vi "New Report Schema and Table Create.vi"(8 "error in":errorcluster, 11 "Schema":string="eDCU_LTT_RESULTS") -> (0 "error out":errorcluster)   [LabVIEW 2023]
uses:
  Database/SQL Public VI/Control/DB Options.ctl
  Database/Database.lvclass
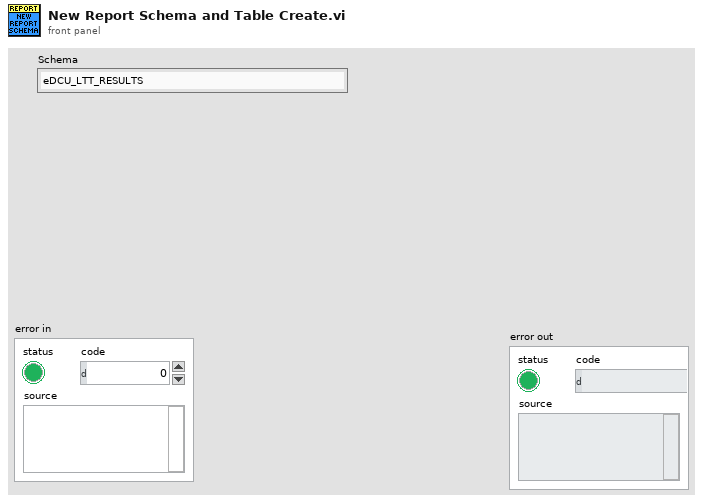
[diagram p1: front panel]
types:
  T1 = typedef "HardwareAbstractionLayer_LVOOP.lvlib/Database.lvclass/DB Options.ctl" = enum16{"Init", "Select Data", "Insert Data", "Update Data", "Delete Data", "Execute Query", "Create Schema", "Create Table", "List Tables", "List Columns", "Close"}
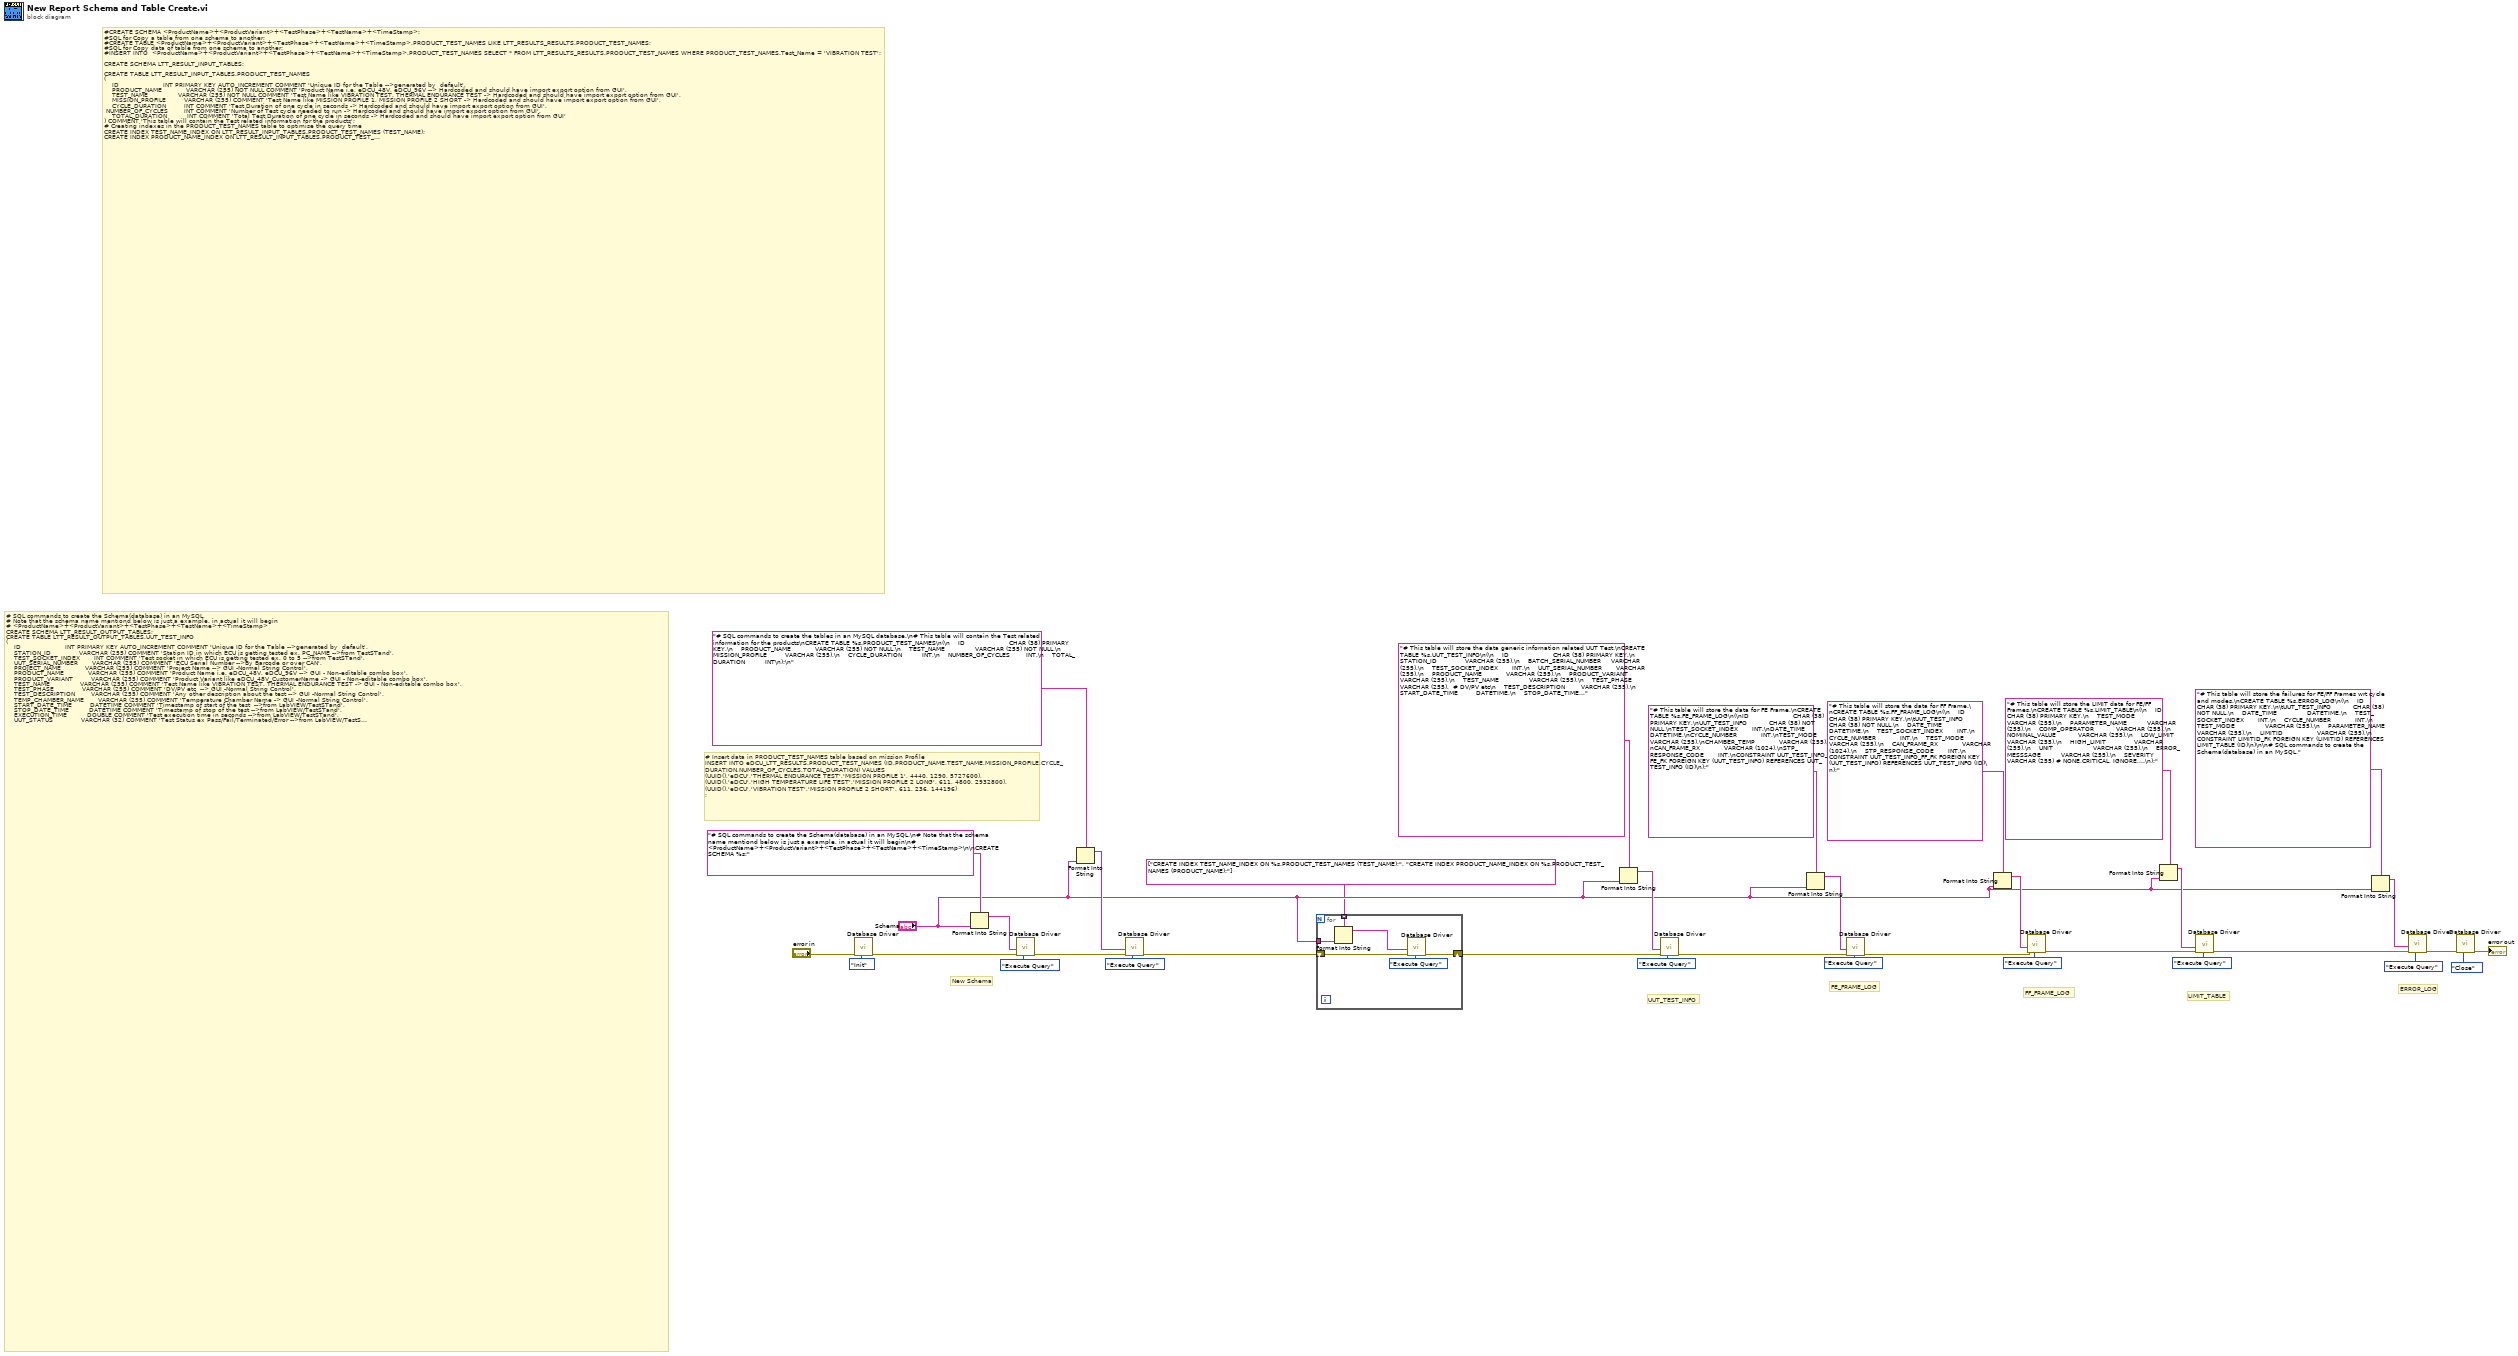
[diagram p0: block diagram]
diagram:
  # "# SQL commands to create the Schema(database) in an MySQL.\n# Note that the schema name mentiond below is just a example, in actual it will begin\n# <ProductName>+<ProductVariant>+<TestPhase>+<TestName>+<TimeStamp>\nCREATE SCHEMA LTT_RESULT_OUTPUT_TABLES;\nCREATE TABLE LTT_RESULT_OUTPUT_TABLES.UUT_TEST_INFO\n(\n    ID                      INT PRIMARY KEY AUTO_INCREMENT COMMENT 'Unique ID for the Table -->generated by  default',\n    STATION_ID              VARCHAR (255) COMMENT 'Station ID in which ECU is getting tested ex. PC_NAME -->from TestSTand',\n    TEST_SOCKET_INDEX       INT COMMENT 'Test socket in which ECU is getting tested ex. 0 to 5 -->from TestSTand',\n    UUT_SERIAL_NUMBER       VARCHAR (255) COMMENT 'ECU Serial Number -->By Barcode or over CAN',\n    PROJECT_NAME            VARCHAR (255) COMMENT 'Project Name --> GUI -Normal String Control',\n    PRODUCT_NAME            VARCHAR (255) COMMENT 'Product Name i.e. eDCU_48V, eDCU_96V --> GUI - Non-editable combo box',\n    PRODUCT_VARIANT         VARCHAR (255) COMMENT 'Product Variant like eDCU_48V_CustomerName -> GUI - Non-editable combo box',\n    TEST_NAME               VARCHAR (255) COMMENT 'Test Name like VIBRATION TEST, THERMAL ENDURANCE TEST -> GUI - Non-editable combo box',\n    TEST_PHASE              VARCHAR (255) COMMENT 'DV/PV etc  --> GUI -Normal String Control',\n    TEST_DESCRIPTION        VARCHAR (255) COMMENT 'Any other description about the test --> GUI -Normal String Control',\n    TEMP_CHAMBER_NAME       VARCHAR (255) COMMENT 'Temperature Chamber Name -> GUI -Normal String Control',\n    START_DATE_TIME         DATETIME COMMENT 'Timestamp of start of the test  -->from LabVIEW/TestSTand',\n    STOP_DATE_TIME          DATETIME COMMENT 'Timestamp of stop of the test -->from LabVIEW/TestSTand',\n    EXECUTION_TIME          DOUBLE COMMENT 'Test execution time in seconds -->from LabVIEW/TestSTand',\n    UUT_STATUS              VARCHAR (32) COMMENT 'Test Status ex Pass/Fail/Terminated/Error -->from LabVIEW/TestSTand',\n    UUT_ERROR_CODE          INT COMMENT 'Error code in case of any error -->from LabVIEW/TestSTand',\n    UUT_ERROR_MESSAGE       VARCHAR (255) COMMENT 'Error Description in case of any error -->from LabVIEW/TestSTand'\n) COMMENT 'This table will store the data generic infornation related UUT Test';\n \nCREATE TABLE LTT_RESULT_OUTPUT_TABLES.FE_FRAME_LOG\n(\n    ID                      INT PRIMARY KEY AUTO_INCREMENT COMMENT 'Unique ID for the Table -->generated by  default',\n\tUUT_TEST_INFO           INT NOT NULL COMMENT 'ID from UUT_TEST_INFO table for that perticular test --> MySQL DB',\n    TEST_SOCKET_INDEX       INT COMMENT 'Test socket in which ECU is getting tested ex. 0 to 5 -->from TestSTand',\n    DATE_TIME               DATETIME COMMENT 'Timestamp when the Frame is received -->from LabVIEW/TestSTand',\n    CYCLE_NUMBER            INT COMMENT 'Current Test Cycle Number of Mission Profile -->from LabVIEW/TestSTand',\n    TEST_MODE               VARCHAR (255) COMMENT 'Current Test Mode of Mission Profile -->from LabVIEW/TestSTand',\n    CHAMBER_TEMP            VARCHAR (255) COMMENT 'Current Temperature of Chamber -->from LabVIEW/TestSTand',\n    CAN_FRAME_RX            VARCHAR (1024) COMMENT 'Raw CAN Frame received over STP -->from LabVIEW/TestSTand',\n    STP_RESPONSE_CODE       INT COMMENT 'STP Response code or Status  received over STP -->from LabVIEW/TestSTand',\n    CONSTRAINT UUT_TEST_INFO_FE_FK FOREIGN KEY (UUT_TEST_INFO) REFERENCES UUT_TEST_INFO (ID)\n) COMMENT 'This table will store the data for FE Frame';\n\n\nCREATE TABLE LTT_RESULT_OUTPUT_TABLES.FF_FRAME_LOG\n(\n    ID                      INT PRIMARY KEY AUTO_INCREMENT COMMENT 'Unique ID for the Table -->generated by  default',\n\tUUT_TEST_INFO           INT NOT NULL COMMENT 'ID from UUT_TEST_INFO table for that perticular test --> MySQL DB',\n\tTEST_SOCKET_INDEX       INT COMMENT 'Test socket in which ECU is getting tested ex. 0 to 5 -->from TestSTand',\n    DATE_TIME               DATETIME COMMENT 'Timestamp when the Frame is received -->from LabVIEW/TestSTand',\n    CYCLE_NUMBER            INT COMMENT 'Current Test Cycle Number of Mission Profile -->from LabVIEW/TestSTand',\n    TEST_MODE               VARCHAR (255) COMMENT 'Current Test Mode of Mission Profile -->from LabVIEW/TestSTand',\n    CHAMBER_TEMP            VARCHAR (255) COMMENT 'Current Temperature of Chamber -->from LabVIEW/TestSTand',\n    CAN_FRAME_RX            VARCHAR (1024) COMMENT 'Raw CAN Frame received over STP -->from LabVIEW/TestSTand',\n    STP_RESPONSE_CODE       INT COMMENT 'STP Response code or Status  received over STP -->from LabVIEW/TestSTand',\n    CONSTRAINT UUT_TEST_INFO_FF_FK FOREIGN KEY (UUT_TEST_INFO) REFERENCES UUT_TEST_INFO (ID)\n) COMMENT 'This table will store the data for FF Frame';\n\nCREATE TABLE LTT_RESULT_OUTPUT_TABLES.LIMIT_TABLE\n(\n    ID                      INT PRIMARY KEY AUTO_INCREMENT COMMENT 'Unique ID for the Table -->generated by  default',\n\tPRODUCT_NAME            VARCHAR (255) COMMENT 'Product Name i.e. eDCU_48V, eDCU_96V --> Hardcoded and should have import export option from GUI',\n    PRODUCT_VARIANT         VARCHAR (255) COMMENT 'Product Variant like eDCU_48V_CustomerName  --> Hardcoded and should have import export option from GUI',\n    TEST_MODE               VARCHAR (255) COMMENT 'Test Mode for which this limit is applicable  --> Hardcoded and should have import export option from GUI',\n    PARAMETER_NAME          VARCHAR (255) COMMENT 'Name of parameter for which this limit is applicable  --> Hardcoded and should have import export option from GUI',\n    COMPARISON_TYPE         VARCHAR (255) COMMENT 'Type of comparison like EQ(for EqualTo) OR GELE(for Greater than Equalto, Less than Equal to) --> Hardcoded and should have import export option from GUI',\n\tLOW_LIMIT               VARCHAR (255) COMMENT 'Low Limit for the Parameter OR Equal Value for the Parameter --> Hardcoded and should have import export option from GUI',\n    HIGH_LIMIT              VARCHAR (255) COMMENT 'Low Limit for the Parameter OR Equal Value for the Parameter --> Hardcoded and should have import export option from GUI',\n    UNIT                    VARCHAR (255) COMMENT 'Unit of  the Parameter --> Hardcoded and should have import export option from GUI',\n    ERROR_MESSSAGE          VARCHAR (255) COMMENT 'Error Message for the Parameter if it is out of range --> Hardcoded and should have import export option from GUI',\n    SEVERITY                VARCHAR (255) COMMENT 'Severity of the Parameter like NONE,CRITICAL, IGNORE, etc --> Hardcoded and should have import export option from GUI'\n) COMMENT 'This table will store the LIMIT data for FE/FF Frames';\n\nCREATE TABLE LTT_RESULT_OUTPUT_TABLES.ERROR_LOG\n(\n    ID                      INT PRIMARY KEY AUTO_INCREMENT COMMENT 'Unique ID for the Table -->generated by  default',\n\tUUT_TEST_INFO           INT NOT NULL COMMENT 'ID from UUT_TEST_INFO table for that perticular test --> MySQL DB',\n    TEST_SOCKET_INDEX       INT COMMENT 'Test socket in which ECU is getting tested ex. 0 to 5 -->from TestSTand',\n    DATE_TIME               DATETIME COMMENT 'Timestamp when the Frame is received -->from LabVIEW/TestSTand',\n    CYCLE_NUMBER            INT COMMENT 'Current Test Cycle Number of Mission Profile -->from LabVIEW/TestSTand',\n    TEST_MODE               VARCHAR (255) COMMENT 'Current Test Mode of Mission Profile -->from LabVIEW/TestSTand',\n    PARAMETER_NAME          VARCHAR (255) COMMENT 'Name of the Test Parameter which is out of limit -->from LabVIEW/TestSTand',\n    LIMITID                 INT NOT NULL COMMENT 'ID from LIMIT_TABLE table for that perticular failure --> MySQL DB',\n    CONSTRAINT LIMITID_FK FOREIGN KEY (LIMITID) REFERENCES LIMIT_TABLE (ID),\n    CONSTRAINT UUT_TEST_INFO_ERROR_LOG_FK FOREIGN KEY (UUT_TEST_INFO) REFERENCES UUT_TEST_INFO (ID)\n) COMMENT 'This table will store the failures for FE/FF Frames wrt cycle and modes';"
  # "#CREATE SCHEMA <ProductName>+<ProductVariant>+<TestPhase>+<TestName>+<TimeStamp>;\n#SQL for Copy a table from one schema to another;\n#CREATE TABLE <ProductName>+<ProductVariant>+<TestPhase>+<TestName>+<TimeStamp>.PRODUCT_TEST_NAMES LIKE LTT_RESULTS_RESULTS.PRODUCT_TEST_NAMES;\n#SQL for Copy data of table from one schema to another;\n#INSERT INTO  <ProductName>+<ProductVariant>+<TestPhase>+<TestName>+<TimeStamp>.PRODUCT_TEST_NAMES SELECT * FROM LTT_RESULTS_RESULTS.PRODUCT_TEST_NAMES WHERE PRODUCT_TEST_NAMES.Test_Name = 'VIBRATION TEST';\n\nCREATE SCHEMA LTT_RESULT_INPUT_TABLES;\n\nCREATE TABLE LTT_RESULT_INPUT_TABLES.PRODUCT_TEST_NAMES\n(\n    ID                      INT PRIMARY KEY AUTO_INCREMENT COMMENT 'Unique ID for the Table -->generated by  default',\n    PRODUCT_NAME            VARCHAR (255) NOT NULL COMMENT 'Product Name i.e. eDCU_48V, eDCU_96V --> Hardcoded and should have import export option from GUI',\n    TEST_NAME               VARCHAR (255) NOT NULL COMMENT 'Test Name like VIBRATION TEST, THERMAL ENDURANCE TEST -> Hardcoded and should have import export option from GUI',\n    MISSION_PROFILE         VARCHAR (255) COMMENT 'Test Name like MISSION PROFILE 1, MISSION PROFILE 2 SHORT -> Hardcoded and should have import export option from GUI',\n    CYCLE_DURATION\t        INT COMMENT 'Test Duration of one cycle in seconds -> Hardcoded and should have import export option from GUI',\n\tNUMBER_OF_CYCLES        INT COMMENT 'Number of Test cycle needed to run -> Hardcoded and should have import export option from GUI',\n    TOTAL_DURATION          INT\tCOMMENT 'Total Test Duration of one cycle in seconds -> Hardcoded and should have import export option from GUI'\n) COMMENT 'This table will contain the Test related information for the products';\n# Creating indexes in the PRODUCT_TEST_NAMES table to optimise the query time\nCREATE INDEX TEST_NAME_INDEX ON LTT_RESULT_INPUT_TABLES.PRODUCT_TEST_NAMES (TEST_NAME);\nCREATE INDEX PRODUCT_NAME_INDEX ON LTT_RESULT_INPUT_TABLES.PRODUCT_TEST_NAMES (PRODUCT_NAME);\n# Insert data in PRODUCT_TEST_NAMES table based on mission Profile\nINSERT INTO LTT_RESULT_INPUT_TABLES.PRODUCT_TEST_NAMES (PRODUCT_NAME,TEST_NAME,MISSION_PROFILE,CYCLE_DURATION,NUMBER_OF_CYCLES,TOTAL_DURATION) VALUES \n('eDCU','THERMAL ENDURANCE TEST','MISSION PROFILE 1', 4440, 1290, 5727600),\n('eDCU','HIGH TEMPERATURE LIFE TEST','MISSION PROFILE 2 LONG', 611, 4800, 2932800),\n('eDCU','VIBRATION TEST','MISSION PROFILE 2 SHORT', 611, 236, 144196)\n;\n\nCREATE TABLE LTT_RESULT_INPUT_TABLES.FE_FRAME_DETAILS\n(\n    ID                      INT PRIMARY KEY AUTO_INCREMENT COMMENT 'Unique ID for the Table -->generated by  default',\n    PRODUCT_NAME            VARCHAR (255) COMMENT 'Product Name i.e. eDCU_48V, eDCU_96V --> GUI - Non-editable combo box',\n    PRODUCT_VARIANT         VARCHAR (255) COMMENT 'Product Variant like eDCU_48V_CustomerName -> GUI - Non-editable combo box',\n    PARAMETER_NAME          VARCHAR (255) COMMENT 'Name of parameter in FE Frame  --> Hardcoded and should have import export option from GUI',\n    OFFSET_NUM\t\t\t\tINT COMMENT 'Offset Number of the Parameter in Return Data --> Hardcoded and should have import export option from GUI',\n    NB_BYTES\t\t\t\tINT\tCOMMENT 'Number of Bytes for the Parameter in Return Data --> Hardcoded and should have import export option from GUI',\n    CONVERSION_FORMULA      VARCHAR (255) COMMENT 'Conversion formula for the parameter ex. (x-32768)/16, optional --> Hardcoded and should have import export option from GUI'\n) COMMENT 'This table will store the details of FE Frames';\n\nCREATE TABLE LTT_RESULT_INPUT_TABLES.FF_FRAME_DETAILS\n(\n    ID                      INT PRIMARY KEY AUTO_INCREMENT COMMENT 'Unique ID for the Table -->generated by  default',\n    PRODUCT_NAME            VARCHAR (255) COMMENT 'Product Name i.e. eDCU_48V, eDCU_96V --> GUI - Non-editable combo box',\n    PRODUCT_VARIANT         VARCHAR (255) COMMENT 'Product Variant like eDCU_48V_CustomerName -> GUI - Non-editable combo box',\n    PARAMETER_NAME          VARCHAR (255) COMMENT 'Name of parameter in FE Frame  --> Hardcoded and should have import export option from GUI',\n    OFFSET_NUM\t\t\t\tINT COMMENT 'Offset Number of the Parameter in Return Data --> Hardcoded and should have import export option from GUI',\n    NB_BYTES\t\t\t\tINT\tCOMMENT 'Number of Bytes for the Parameter in Return Data --> Hardcoded and should have import export option from GUI',\n    CONVERSION_FORMULA      VARCHAR (255) COMMENT 'Conversion formula for the parameter ex. (x-32768)/16, optional --> Hardcoded and should have import export option from GUI'\n) COMMENT 'This table will store the details of FF Frames';\n\n\nCREATE TABLE LTT_RESULT_INPUT_TABLES.LIMIT_TABLE\n(\n    ID                      INT PRIMARY KEY AUTO_INCREMENT COMMENT 'Unique ID for the Table -->generated by  default',\n\tPRODUCT_NAME            VARCHAR (255) COMMENT 'Product Name i.e. eDCU_48V, eDCU_96V --> Hardcoded and should have import export option from GUI',\n    PRODUCT_VARIANT         VARCHAR (255) COMMENT 'Product Variant like eDCU_48V_CustomerName  --> Hardcoded and should have import export option from GUI',\n    TEST_MODE               VARCHAR (255) COMMENT 'Test Mode for which this limit is applicable  --> Hardcoded and should have import export option from GUI',\n    PARAMETER_NAME          VARCHAR (255) COMMENT 'Name of parameter for which this limit is applicable  --> Hardcoded and should have import export option from GUI',\n    COMPARISON_TYPE         VARCHAR (255) COMMENT 'Type of comparison like EQ(for EqualTo) OR GELE(for Greater than Equalto, Less than Equal to) --> Hardcoded and should have import export option from GUI',\n\tLOW_LIMIT               VARCHAR (255) COMMENT 'Low Limit for the Parameter OR Equal Value for the Parameter --> Hardcoded and should have import export option from GUI',\n    HIGH_LIMIT              VARCHAR (255) COMMENT 'Low Limit for the Parameter OR Equal Value for the Parameter --> Hardcoded and should have import export option from GUI',\n    UNIT                    VARCHAR (255) COMMENT 'Unit of  the Parameter --> Hardcoded and should have import export option from GUI',\n    ERROR_MESSSAGE          VARCHAR (255) COMMENT 'Error Message for the Parameter if it is out of range --> Hardcoded and should have import export option from GUI',\n    SEVERITY                VARCHAR (255) COMMENT 'Severity of the Parameter like NONE,CRITICAL, IGNORE, etc --> Hardcoded and should have import export option from GUI'\n) COMMENT 'This table will store the LIMIT data for FE/FF Frames';"
  # "# Insert data in PRODUCT_TEST_NAMES table based on mission Profile\nINSERT INTO eDCU_LTT_RESULTS.PRODUCT_TEST_NAMES (ID,PRODUCT_NAME,TEST_NAME,MISSION_PROFILE,CYCLE_DURATION,NUMBER_OF_CYCLES,TOTAL_DURATION) VALUES \n(UUID(),'eDCU','THERMAL ENDURANCE TEST','MISSION PROFILE 1', 4440, 1290, 5727600),\n(UUID(),'eDCU','HIGH TEMPERATURE LIFE TEST','MISSION PROFILE 2 LONG', 611, 4800, 2932800),\n(UUID(),'eDCU','VIBRATION TEST','MISSION PROFILE 2 SHORT', 611, 236, 144196)\n;"
  # "ERROR_LOG"
  # "LIMIT_TABLE"
  # "FF_FRAME_LOG"
  # "FE_FRAME_LOG"
  # "UUT_TEST_INFO"
  # "New Schema"
  n1 = call "Database Driver.vi"("Options"=DB_Options."Init", "error in"="error in") -> ("error out"=w34:errorcluster)  [unwired: 6 in, 3 out]
  n2 = Format Into String(format string="# SQL commands to create the Schema(database) in an MySQL.\n# Note that the schema name mentiond below is just a example, in actual it will begin\n# <ProductName>+<ProductVariant>+<TestPhase>+<TestName>+<TimeStamp>\n\nCREATE SCHEMA %s;", "Schema") -> (resulting string=w31:string)  [unwired: 2 in, 1 out]
  n3 = call "Database Driver.vi"("Options"=DB_Options."Execute Query", "error in"=w34, "SQL query"=w31) -> ("error out"=w7:errorcluster)  [unwired: 5 in, 3 out]
  n4 = Format Into String(format string="# SQL commands to create the tables in an MySQL database.\n# This table will contain the Test related information for the products\nCREATE TABLE %s.PRODUCT_TEST_NAMES\n(\n    ID                      CHAR (38) PRIMARY KEY,\n    PRODUCT_NAME            VARCHAR (255) NOT NULL,\n    TEST_NAME               VARCHAR (255) NOT NULL,\n    MISSION_PROFILE         VARCHAR (255),\n    CYCLE_DURATION          INT,\n    NUMBER_OF_CYCLES        INT,\n    TOTAL_DURATION          INT\n);\n", "Schema") -> (resulting string=w6:string)  [unwired: 2 in, 1 out]
  n5 = call "Database Driver.vi"("Options"=DB_Options."Execute Query", "error in"=w7, "SQL query"=w6) -> ("error out"=w4:errorcluster)  [unwired: 5 in, 3 out]
  n6 = for {
    tunnel: "Schema" -> [w38]
    tunnel: string[] ["CREATE INDEX TEST_NAME_INDEX ON %s.PRODUCT_TEST_NAMES (TEST_NAME);", "CREATE INDEX PRODUCT_NAME_INDEX ON %s.PRODUCT_TEST_NAMES (PRODUCT_NAME);"] -> [w37] mode=indexing
    shift-right: [w41] -> w3
    shift-left: w4 -> [w42]
    n7 = Format Into String(format string=w37, w38) -> (resulting string=w40:string)  [unwired: 2 in, 1 out]
    n8 = call "Database Driver.vi"("Options"=DB_Options."Execute Query", "error in"=w42, "SQL query"=w40) -> ("error out"=w41:errorcluster)  [unwired: 5 in, 3 out]
  }
  n9 = Format Into String(format string="# This table will store the data generic infornation related UUT Test.\nCREATE TABLE %s.UUT_TEST_INFO\n(\n    ID                      CHAR (38) PRIMARY KEY,\n    STATION_ID              VARCHAR (255),\n    BATCH_SERIAL_NUMBER     VARCHAR (255),\n    TEST_SOCKET_INDEX       INT,\n    UUT_SERIAL_NUMBER       VARCHAR (255),\n    PRODUCT_NAME            VARCHAR (255),\n    PRODUCT_VARIANT         VARCHAR (255),\n    TEST_NAME               VARCHAR (255),\n    TEST_PHASE              VARCHAR (255),  # DV/PV etc\n    TEST_DESCRIPTION        VARCHAR (255),\n    START_DATE_TIME         DATETIME,\n    STOP_DATE_TIME          DATETIME,\n    EXECUTION_TIME          DOUBLE,    \n    UUT_STATUS              VARCHAR (32),\n    UUT_ERROR_CODE          INT,\n    UUT_ERROR_MESSAGE       VARCHAR (255),\n    TEMP_CHAMBER_NAME       VARCHAR (255)\n);", "Schema") -> (resulting string=w17:string)  [unwired: 2 in, 1 out]
  n10 = call "Database Driver.vi"("Options"=DB_Options."Execute Query", "error in"=w3, "SQL query"=w17) -> ("error out"=w33:errorcluster)  [unwired: 5 in, 3 out]
  n11 = Format Into String(format string="# This table will store the data for FE Frame.\nCREATE TABLE %s.FE_FRAME_LOG\n(\nID                      CHAR (38) PRIMARY KEY,\nUUT_TEST_INFO           CHAR (38) NOT NULL,\nTEST_SOCKET_INDEX       INT,\nDATE_TIME               DATETIME,\nCYCLE_NUMBER            INT,\nTEST_MODE               VARCHAR (255),\nCHAMBER_TEMP            VARCHAR (255),\nCAN_FRAME_RX            VARCHAR (1024),\nSTP_RESPONSE_CODE       INT,\nCONSTRAINT UUT_TEST_INFO_FE_FK FOREIGN KEY (UUT_TEST_INFO) REFERENCES UUT_TEST_INFO (ID)\n);" ("SQL query"), "Schema") -> (resulting string=w15:string)  [unwired: 2 in, 1 out]
  n12 = call "Database Driver.vi"("Options"=DB_Options."Execute Query", "error in"=w33, "SQL query"=w15) -> ("error out"=w26:errorcluster)  [unwired: 5 in, 3 out]
  n13 = Format Into String(format string="# This table will store the data for FF Frame.\nCREATE TABLE %s.FF_FRAME_LOG\n(\n    ID                      CHAR (38) PRIMARY KEY,\n\tUUT_TEST_INFO           CHAR (38) NOT NULL,\n    DATE_TIME               DATETIME,\n    TEST_SOCKET_INDEX       INT,\n    CYCLE_NUMBER            INT,\n    TEST_MODE               VARCHAR (255),\n    CAN_FRAME_RX            VARCHAR (1024),\n    STP_RESPONSE_CODE       INT,\n    CONSTRAINT UUT_TEST_INFO_FF_FK FOREIGN KEY (UUT_TEST_INFO) REFERENCES UUT_TEST_INFO (ID)\n);" ("SQL query"), "Schema") -> (resulting string=w13:string)  [unwired: 2 in, 1 out]
  n14 = call "Database Driver.vi"("Options"=DB_Options."Execute Query", "error in"=w26, "SQL query"=w13) -> ("error out"=w22:errorcluster)  [unwired: 5 in, 3 out]
  n15 = Format Into String(format string="# This table will store the LIMIT data for FE/FF Frames.\nCREATE TABLE %s.LIMIT_TABLE\n(\n    ID                      CHAR (38) PRIMARY KEY,\n    TEST_MODE               VARCHAR (255),\n    PARAMETER_NAME          VARCHAR (255),\n    COMP_OPERATOR           VARCHAR (255),\n    NOMINAL_VALUE           VARCHAR (255),\n    LOW_LIMIT               VARCHAR (255),\n    HIGH_LIMIT              VARCHAR (255),\n    UNIT                    VARCHAR (255),\n    ERROR_MESSSAGE          VARCHAR (255),\n    SEVERITY                VARCHAR (255) # NONE,CRITICAL, IGNORE,...\n);" ("SQL query"), "Schema") -> (resulting string=w11:string)  [unwired: 2 in, 1 out]
  n16 = call "Database Driver.vi"("Options"=DB_Options."Execute Query", "error in"=w22, "SQL query"=w11) -> ("error out"=w19:errorcluster)  [unwired: 5 in, 3 out]
  n17 = Format Into String(format string="# This table will store the failures for FE/FF Frames wrt cycle and modes.\nCREATE TABLE %s.ERROR_LOG\n(\n    ID                      CHAR (38) PRIMARY KEY,\n\tUUT_TEST_INFO           CHAR (38) NOT NULL,\n    DATE_TIME               DATETIME,\n    TEST_SOCKET_INDEX       INT,\n    CYCLE_NUMBER            INT,\n    TEST_MODE               VARCHAR (255),\n    PARAMETER_NAME          VARCHAR (255),\n    LIMITID                 VARCHAR (255),\n    CONSTRAINT LIMITID_FK FOREIGN KEY (LIMITID) REFERENCES LIMIT_TABLE (ID)\n)\n\n# SQL commands to create the Schema(database) in an MySQL." ("SQL query"), "Schema") -> (resulting string=w9:string)  [unwired: 2 in, 1 out]
  n18 = call "Database Driver.vi"("Options"=DB_Options."Execute Query", "error in"=w19, "SQL query"=w9) -> ("error out"=w24:errorcluster)  [unwired: 5 in, 3 out]
  n19 = call "Database Driver.vi"("Options"=DB_Options."Close", "error in"=w24) -> ("error out"=→"error out":errorcluster)  [unwired: 6 in, 3 out]
